vi "删除历史图片和数据.vi"() -> ()   [LabVIEW 2014]
uses:
  Controls/MsgAction.ctl
  Global.vi
panel:
  out "删除图片进度条":u8(slide) scale=0.0..100.0
  out "文件名":string[](array[string])
  out "相隔天数":dbl
  # "删除历史图片和数据中，请耐心等待！\n点“取消”按钮，暂时不删除图片和数据！"
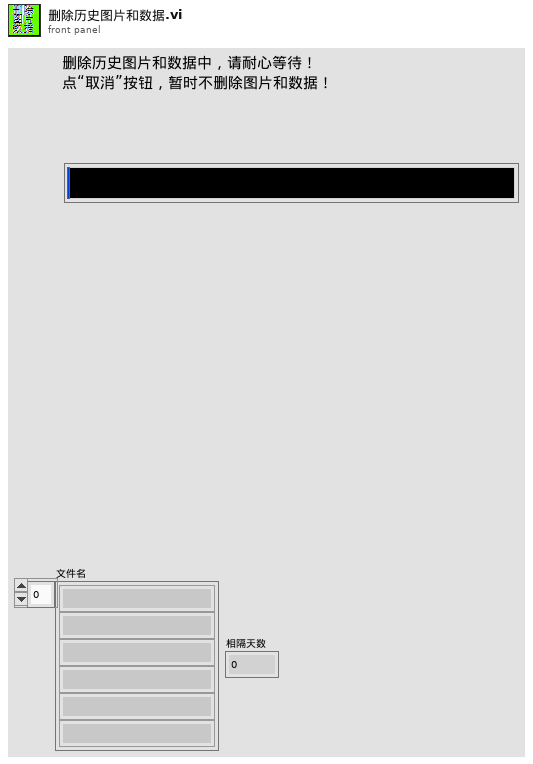
[diagram p1: front panel]
types:
  T1 = enum16{"7天", "30天", "永远", "500张", "1000张", "10000张"}
  T2 = typedef "MsgAction.ctl" = enum16{"初始化", "添加消息", "区分结果添加消息", "清空消息", "获取消息"}
  T3 = typedef "OtherSpec.ctl" = cluster{"数值类规格":T4, "勾选规格":T5}
  T4 = typedef "数值类规格.ctl" = cluster{"数据保存容量":enum16{"7天", "30天", "永远"}, "图片保存容量":enum16{"7天", "30天", "永远", "500张", "1000张", "10000张"}}
  T5 = typedef "勾选规格.ctl" = cluster{"保存不良图片":bool, "保存合格图片":bool, "保存数据?":bool, "每次开程式自动删除图片数据":bool, "显示曲线图":bool, "测试不良时蜂鸣器响":bool}
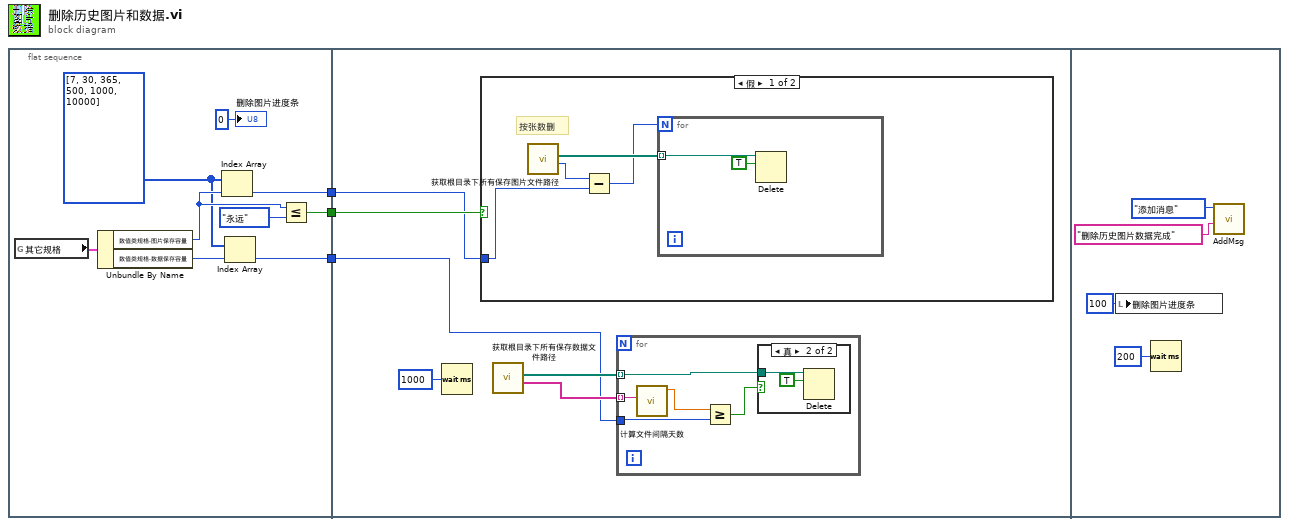
[diagram p0: block diagram]
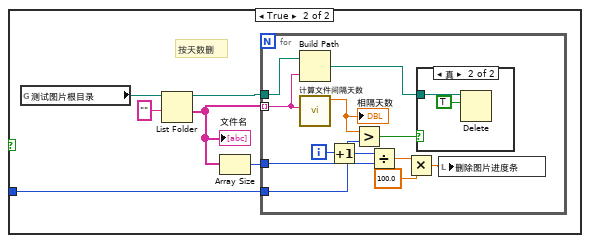
[diagram p2: hidden frame]
diagram:
  n1 = flat-sequence {
    tunnel: [w5] -> w3
    tunnel: [w6] -> w2
    tunnel: [w4] -> w1
    tunnel: w3 -> [w15]
    tunnel: w2 -> [w14]
    tunnel: w1 -> [w13]
    frame #0 {
      w8 = i32[] [7, 30, 365, 500, 1000, 10000] ("数组")
      n2 = global read "Global.vi" "其它规格"() -> (w7:T3)
      n3 = Unbundle By Name(w7) -> ("数值类规格.图片保存容量"=w10:T1, "数值类规格.数据保存容量"=w9:enum16{"7天", "30天", "永远"})
      n4 = Index Array(array=w8, index=w10) -> (element=w4:i32)
      n5 = Index Array(array=w8, index=w9) -> (element=w6:i32)
      n6 = Less Or Equal?(x=w10, y=T1."永远") -> (x <= y?=w5:bool)
      "删除图片进度条" <- u8 0 ("删除图片进度条")
    }
    frame #1 {
      n7 = Wait (ms)(milliseconds to wait=u32 1000 ("等待时间（毫秒）")) -> ()  [unwired: 1 out]
      n8 = case shown="假" w15 {
        tunnel: w13 -> [w20 w25]
        frame False {
          # "按张数删"
          n9 = call "获取根目录下所有保存图片文件路径.vi"() -> ("图片张数"=w21:i32, "所有图片路径"=w22:path[])  [unwired: 10 in]
          n10 = Subtract(x=w21, y=w20) -> (x-y=w19:i32)
          n11 = for {
            N: w19 -> [_]
            tunnel: w22 -> [w24] mode=indexing
            n12 = Delete(path (use dialog)=w24, entire hierarchy (F)=TRUE ("整个层次结构(F)")) -> ()  [unwired: 3 in, 3 out]
          }
        }
        frame True {
          # "按天数删"
          n13 = global read "Global.vi" "测试图片根目录"() -> (w30:path)
          n14 = List Folder ("罗列文件夹")(path=w30, pattern="" ("模式")) -> (path out=w29:path, folder names=w27:string[])  [unwired: 2 in, 2 out]
          "文件名" <- w27
          n15 = Array Size(array=w27) -> (size(s)=w26:i32)
          n16 = for {
            tunnel: w29 -> [w42]
            tunnel: w27 -> [w41] mode=indexing
            tunnel: w25 -> [w39]
            tunnel: w26 -> [w36]
            i -> [w37]
            n17 = Build Path(base path=w42, name or relative path=w41) -> (appended path=w40:path)
            n18 = call "计算文件间隔天数.vi"("字符串"=w41) -> ("数值"=w31:dbl)  [unwired: 10 in]
            "相隔天数" <- w31
            n19 = Increment(x=w37) -> (x+1=w35:i32)
            n20 = Greater?(x=w31, y=w39) -> (0:w38:bool)
            n21 = Divide(x=w35, y=w36) -> (x/y=w34:dbl)
            n22 = Multiply(x=w34, y=100.0) -> (x*y=w33:dbl)
            n23 = case shown="真" w38 {
              tunnel: w40 -> [_ w44]
              frame False {
              }
              frame True {
                n24 = Delete(path (use dialog)=w44, entire hierarchy (F)=TRUE ("整个层次结构(F)")) -> ()  [unwired: 3 in, 3 out]
              }
            }
            n25 = local write "删除图片进度条"(w33) -> ()
          }
        }
      }
      n26 = call "获取根目录下所有保存数据文件路径.vi"() -> ("文档日期"=w16:string[], "所有存档数据表路径"=w17:path[])  [unwired: 10 in]
      n27 = for {
        tunnel: w17 -> [w49] mode=indexing
        tunnel: w16 -> [w48] mode=indexing
        tunnel: w14 -> [w45]
        n28 = call "计算文件间隔天数.vi"("字符串"=w48) -> ("数值"=w47:dbl)  [unwired: 10 in]
        n29 = Greater Or Equal?(x=w47, y=w45) -> (x >= y?=w46:bool)
        n30 = case shown="真" w46 {
          tunnel: w49 -> [_ w50]
          frame False {
          }
          frame True {
            n31 = Delete(path (use dialog)=w50, entire hierarchy (F)=TRUE ("整个层次结构(F)")) -> ()  [unwired: 3 in, 3 out]
          }
        }
      }
    }
    frame #2 {
      n32 = local write "删除图片进度条"(u8 100 ("删除图片进度条")) -> ()
      n33 = Wait (ms)(milliseconds to wait=u32 200 ("等待时间（毫秒）")) -> ()  [unwired: 1 out]
      n34 = call "AddMsg.vi"("添加消息"="删除历史图片数据完成" ("消息显示"), "消息Action"=MsgAction."添加消息") -> ()  [unwired: 2 in, 1 out]
    }
  }
